vi "Machs1-11-15.vi"(0 "Heizen?Mach1":bool, 1 "Heizen?Mach2":bool, 2 "PIDMach1":T1 {"proportional gain (Kc)" format="%.11g"; "integral gain (Kc*Ts/Ti)" format="%.11g"; "derivative gain (Kc*Td/Ts)" format="%.11g"}, 3 "PIDMach2":T1 {"proportional gain (Kc)" format="%.11g"; "integral gain (Kc*Ts/Ti)" format="%.11g"; "derivative gain (Kc*Td/Ts)" format="%.11g"}, 4 "Umax[V]Mach1":fxp<+/-,16,4> format="%.14g", 5 "Umax[V]Mach2":fxp<+/-,16,4> format="%.14g", 6 "USetp[V]Mach1":fxp<+/-,16,4> format="%.14g", 7 "USetp[V]Mach2":fxp<+/-,16,4> format="%.14g", 10 "Per[us]Mach":u16 caption="Periode Mach [us]", 11 "Mach1maxHigh":u16, 12 "vor der Messung [us]Mach":u16=200, 14 "wie viele Messwerte?Mach":u16, 15 "Mach2High?":bool, 16 "Abstand zwischen Messungen [us]Mach":u16 caption="Abstand zwischen Messungen Mach [us]", 17 "Mach2High":u16) -> (20 "U[V]Mach1":fxp<+/-,16,4> format="%.25g", 21 "U[V]Mach2":fxp<+/-,16,4> format="%.25g", 23 "Mach1maxHigh":u16, 26 "Mach2High?":bool, 27 "Mach2High":u16)   [LabVIEW 2010]
uses:
  <vilib>/eio/EIONode/EIONode.xnode
  <vilib>/rvi/eio/nirviEIOImplementation/nirviEIOImplementation.xnode
  <vilib>/rvi/eio/common/nirviEmuClasses.ctl
  <vilib>/rvi/FXPMathLib/FxpAdd/XNode/nifxpmath_Add.xnode
  <vilib>/rvi/FXPMathLib/FxpAdd/subVIs/nifxpmath_Add_SimConfig.ctl
  <vilib>/fxp/LVFixedPointQuantizationPolicyTypeDef.ctl
  <vilib>/fxp/LVFixedPointOverflowPolicyTypeDef.ctl
  <vilib>/rvi/FXPMathLib/FxpDiv/XNode/nifxpmath_Div.xnode
  <vilib>/rvi/FXPMathLib/FxpDiv/subVIs/nifxpmath_Div_SimConfig.ctl
  <vilib>/rvi/FXPMathLib/FxpMul/XNode/nifxpmath_Multiplier.xnode
  <vilib>/rvi/FXPMathLib/FxpMul/subVIs/nifxpmath_Mul_SimConfig.ctl
  <vilib>/rvi/FXPMathLib/FxpSqrt/XNode/nifxpmath_Sqrt.xnode
  <vilib>/rvi/FXPMathLib/FxpSqrt/subVIs/nifxpmath_Sqrt_SimConfig.ctl
  <vilib>/rvi/FXPMathLib/FxpConvert/XNode/nifxpmath_Convert.xnode
  <vilib>/rvi/FXPMathLib/FxpConvert/subVIs/nifxpmath_Convert_SimConfig.ctl
  <vilib>/addons/control/pid/fpga.llb/XNode/niFpgaPID.xnode
  <vilib>/rvi/eio/common/nirviEmuTemplateMethod_noerrors.vi
  <vilib>/rvi/FXPMathLib/FxpAdd/simVIs/DllFxpAddTemp_sub.vi
  <vilib>/rvi/FXPMathLib/FxpDiv/simVIs/DllFxpDivTemp_sub.vi
  <vilib>/rvi/FXPMathLib/FxpMul/simVIs/DllFxpMulTemp_sub.vi
  <vilib>/rvi/FXPMathLib/FxpSqrt/simVIs/DllSqrtTemp_sub.vi
  <vilib>/rvi/FXPMathLib/FxpConvert/simVIs/DllFxpConvertTemp_sub.vi
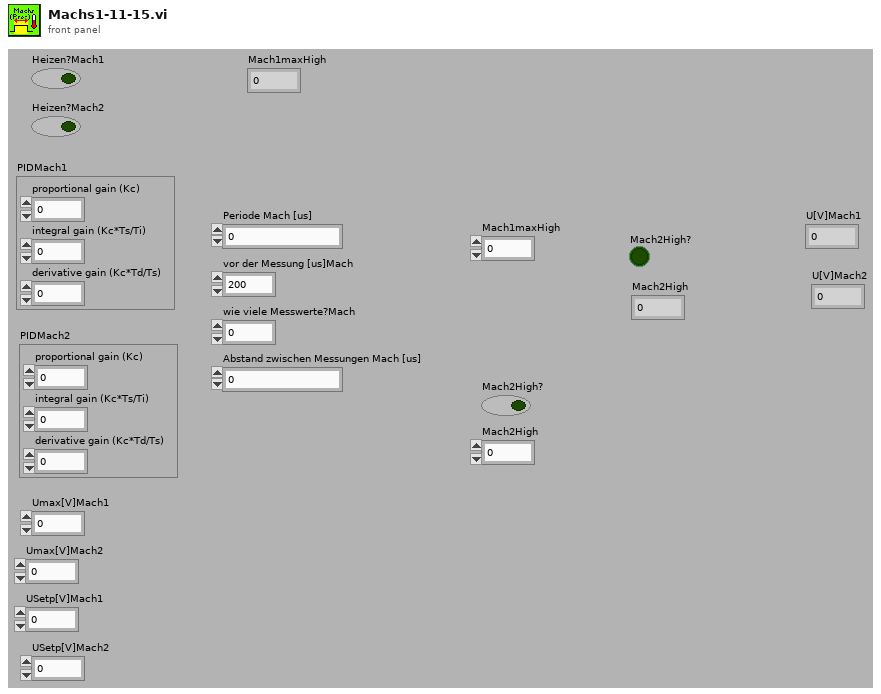
[diagram p1: front panel]
types:
  T1 = cluster{"proportional gain (Kc)":fxp<+/-,16,8>, "integral gain (Kc*Ts/Ti)":fxp<+/-,16,8>, "derivative gain (Kc*Td/Ts)":fxp<+/-,16,8>}
  T2 = cluster{"output high":fxp<+/-,16,4>, "output low":fxp<+/-,16,4>}
  T3 = typedef "nirviEmuClasses.ctl" = enum16{"IO Read", "IO Write", "Method", "Property Read", "Property Write"}
  T4 = cluster{"proportional gain (Kc)":i16, "integral gain (Kc*Ts/Ti)":i16, "derivative gain (Kc*Td/Ts)":i16}
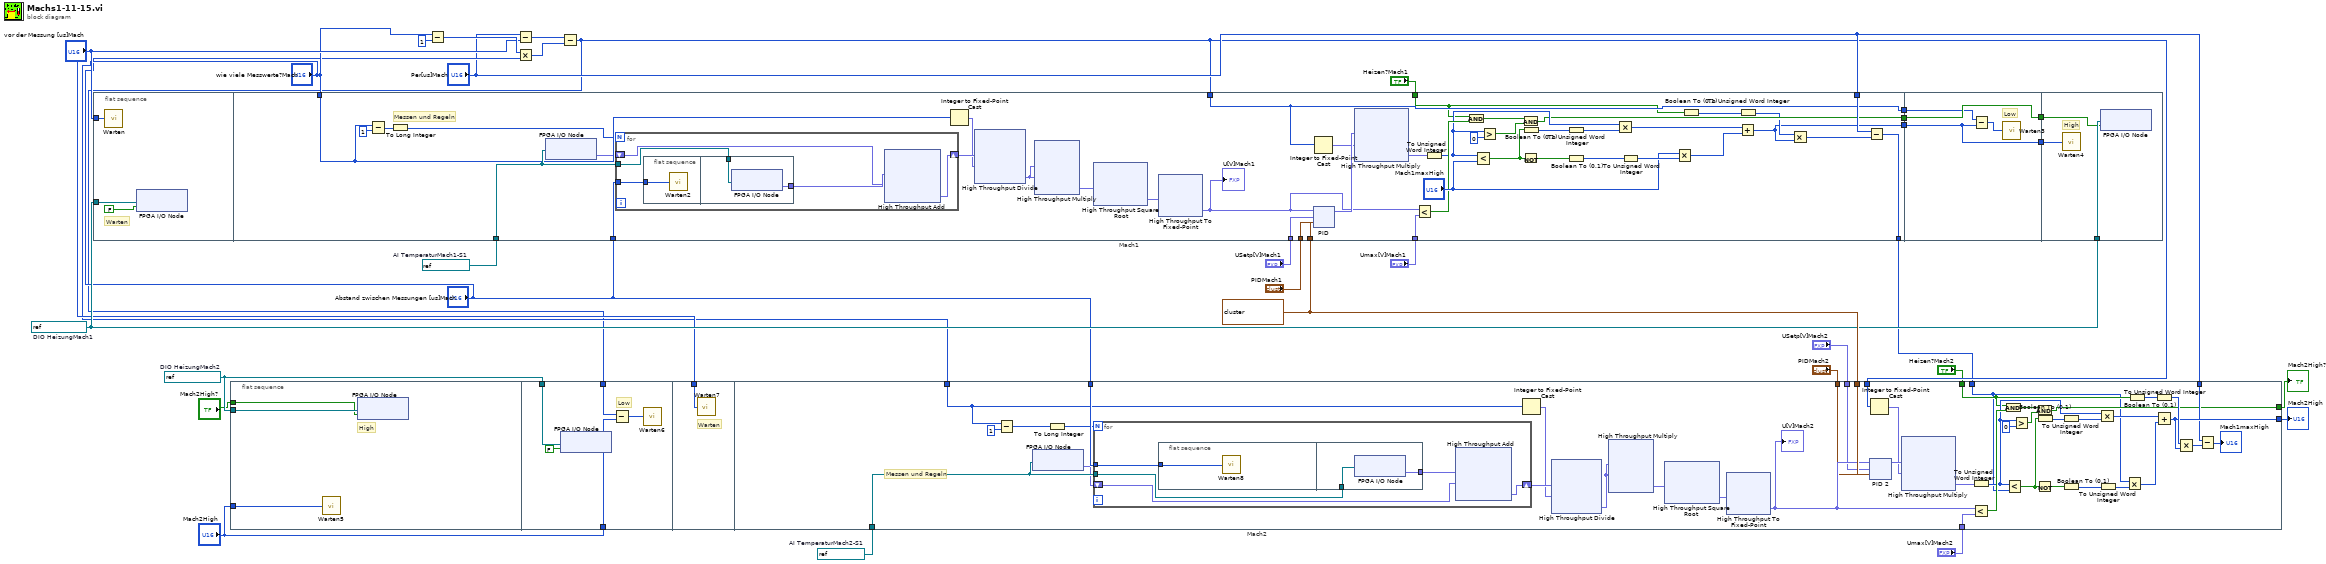
[diagram p0: block diagram]
diagram:
  w23 = refnum<k21> "Mod6/DIO22"  # DIO HeizungMach2
  w24 = refnum<k21> "Mod1/AI4"  # AI TemperaturMach2-S1
  w25 = refnum<k21> "Mod1/AI3"  # AI TemperaturMach1-S1
  w26 = refnum<k21> "Mod6/DIO23"  # DIO HeizungMach1
  w27 = T2 {"output high"=1.0, "output low"=0.0} ("output range")
  n1 = flat-sequence "Mach1" {
    tunnel: "vor der Messung [us]Mach" -> [w35]
    tunnel: w26 -> [w34]
    tunnel: w25 -> [w88]
    tunnel: "Abstand zwischen Messungen [us]Mach" -> [w84]
    tunnel: "wie viele Messwerte?Mach" -> [w86]
    tunnel: "Per[us]Mach" -> [w69]
    tunnel: [w60] -> w32
    tunnel: [w63] -> w31
    tunnel: [w58] -> w30
    tunnel: w10 -> [w58]
    tunnel: w27 -> [w57]
    tunnel: "Umax[V]Mach1" -> [w52]
    tunnel: "USetp[V]Mach1" -> [w51]
    tunnel: "Heizen?Mach1" -> [w50]
    tunnel: "PIDMach1" -> [w49]
    tunnel: [w48] -> w1
    tunnel: [w335] -> w29
    tunnel: w32 -> [w335]
    tunnel: [w336] -> w28
    tunnel: w31 -> [w336]
    tunnel: w30 -> [w334]
    tunnel: w26 -> [w339]
    tunnel: w29 -> [w338]
    tunnel: w28 -> [w337]
    frame #0 {
      # "Warten"
      n2 = call "Warten"("Count(uSec)"=w35) -> ()  [unwired: 1 out]
      n3 = xnode "FPGA I/O Node"("I/O Item"=FALSE, "FPGA I/O In"=w34) -> ()  [unwired: 1 out]
    }
    frame #1 {
      # "Messen und Regeln"
      n4 = Subtract(x=w86, y=u16 1) -> (x-y=w83:u16)
      n5 = To Long Integer(number=w83) -> (32bit integer=w82:i32)
      n6 = xnode "FPGA I/O Node"("FPGA I/O In"=w88) -> ("I/O Item"=w47:fxp<+/-,26,5>)  [unwired: 1 out]
      n7 = for {
        N: w82 -> [_]
        shift-right: [w230] -> w87
        shift-left: w47 -> [w231]
        tunnel: w84 -> [w234]
        tunnel: w88 -> [w233]
        n8 = flat-sequence {
          tunnel: w234 -> [w265]
          tunnel: w233 -> [w267]
          tunnel: [w266] -> w232
          frame #0 {
            n9 = call "Warten2"("Count(uSec)"=w265) -> ()  [unwired: 1 out]
          }
          frame #1 {
            n10 = xnode "FPGA I/O Node"("FPGA I/O In"=w267) -> ("I/O Item"=w266:fxp<+/-,26,5>)  [unwired: 1 out]
          }
        }
        n11 = xnode "High Throughput Add"("x"=w232, "y"=w231) -> ("x+y"=w230:fxp<+/-,32,11>)
      }
      n12 = Integer to Fixed-Point Cast ("Integer in Festkomma umwandeln")(integer=w86) -> (fixed-point=w85:fxp<+/-,8,8>)  [unwired: 1 in]
      n13 = xnode "High Throughput Divide"("x"=w87, "y"=w85) -> ("x/y"=w56:fxp<+/-,16,4>)
      n14 = xnode "High Throughput Multiply"("x"=w56, "y"=w56) -> ("x*y"=w55:fxp<+,32,8>)
      n15 = xnode "High Throughput Square Root"("x"=w55) -> ("sqrt(x)"=w54:fxp<+,16,4>)
      n16 = xnode "High Throughput To Fixed-Point"("x"=w54) -> ("y"=w53:fxp<+/-,16,4>)
      "U[V]Mach1" <- w53
      n17 = xnode ("PID")("process variable"=w53, "setpoint"=w51, "PID gains"=w49, "output range"=w57) -> ("output"=w81:fxp<+/-,16,4>)  [unwired: 1 in]
      n18 = Integer to Fixed-Point Cast ("Integer in Festkomma umwandeln")(integer=w58) -> (fixed-point=w80:fxp<+,16,16>)  [unwired: 1 in]
      n19 = xnode "High Throughput Multiply"("x"=w81, "y"=w80) -> ("x*y"=w79:fxp<+/-,16,16>)
      n20 = Less?(x=w53, y=w52) -> (x < y?=w68:bool)
      n21 = To Unsigned Word Integer(number=w79) -> (unsigned 16bit integer=w67:u16)
      n22 = And(x=w50, y=w68) -> (x .and. y?=w65:bool)
      n23 = Less?(x=w67, y="Mach1maxHigh") -> (x < y?=w74:bool)
      n24 = Greater?(x=w67, y=u16 0) -> (0:w64:bool)
      n25 = And(x=w65, y=w64) -> (x .and. y?=w63:bool)
      n26 = Boolean To (0,1)(Boolean=w74) -> (0, 1=w78:i16)
      n27 = Not(x=w74) -> (.not. x?=w73:bool)
      n28 = To Unsigned Word Integer(number=w78) -> (unsigned 16bit integer=w77:u16)
      n29 = Boolean To (0,1)(Boolean=w73) -> (0, 1=w76:i16)
      n30 = Multiply(x=w67, y=w77) -> (x*y=w71:u16)
      n31 = To Unsigned Word Integer(number=w76) -> (unsigned 16bit integer=w75:u16)
      n32 = Multiply(x="Mach1maxHigh", y=w75) -> (x*y=w70:u16)
      n33 = Boolean To (0,1)(Boolean=w50) -> (0, 1=w62:i16)
      n34 = To Unsigned Word Integer(number=w62) -> (unsigned 16bit integer=w61:u16)
      n35 = Add(x=w71, y=w70) -> (x+y=w60:u16)
      n36 = Multiply(x=w61, y=w60) -> (x*y=w59:u16)
      n37 = Subtract(x=w69, y=w59) -> (x-y=w48:u16)
    }
    frame #2 {
      # "Low"
      n38 = Subtract(x=w334, y=w335) -> (x-y=w333:u16)
      n39 = call "Warten3"("Count(uSec)"=w333) -> ()  [unwired: 1 out]
    }
    frame #3 {
      # "High"
      n40 = call "Warten4"("Count(uSec)"=w338) -> ()  [unwired: 1 out]
      n41 = xnode "FPGA I/O Node"("I/O Item"=w337, "FPGA I/O In"=w339) -> ()  [unwired: 1 out]
    }
  }
  n42 = flat-sequence "Mach2" {
    tunnel: "Mach2High" -> [w351]
    tunnel: w23 -> [w353]
    tunnel: "Mach2High?" -> [w352]
    tunnel: w23 -> [w369]
    tunnel: w10 -> [w367]
    tunnel: "Mach2High" -> [w366]
    tunnel: "vor der Messung [us]Mach" -> [w381]
    tunnel: w24 -> [w423]
    tunnel: "Abstand zwischen Messungen [us]Mach" -> [w424]
    tunnel: "wie viele Messwerte?Mach" -> [w419]
    tunnel: w27 -> [w415]
    tunnel: w10 -> [w400]
    tunnel: [w401] -> w19
    tunnel: "Per[us]Mach" -> [w398]
    tunnel: [w393] -> w20
    tunnel: "USetp[V]Mach2" -> [w388]
    tunnel: "PIDMach2" -> [w387]
    tunnel: "Umax[V]Mach2" -> [w386]
    tunnel: "Heizen?Mach2" -> [w385]
    tunnel: w1 -> [w383]
    frame #0 {
      # "High"
      n43 = call "Warten5"("Count(uSec)"=w351) -> ()  [unwired: 1 out]
      n44 = xnode "FPGA I/O Node"("I/O Item"=w352, "FPGA I/O In"=w353) -> ()  [unwired: 1 out]
    }
    frame #1 {
      # "Low"
      n45 = xnode "FPGA I/O Node"("I/O Item"=FALSE, "FPGA I/O In"=w369) -> ()  [unwired: 1 out]
      n46 = Subtract(x=w367, y=w366) -> (x-y=w365:u16)
      n47 = call "Warten6"("Count(uSec)"=w365) -> ()  [unwired: 1 out]
    }
    frame #2 {
      # "Warten"
      n48 = call "Warten7"("Count(uSec)"=w381) -> ()  [unwired: 1 out]
    }
    frame #3 {
      # "Messen und Regeln"
      n49 = Subtract(x=w419, y=u16 1) -> (x-y=w421:u16)
      n50 = xnode "FPGA I/O Node"("FPGA I/O In"=w423) -> ("I/O Item"=w382:fxp<+/-,26,5>)  [unwired: 1 out]
      n51 = To Long Integer(number=w421) -> (32bit integer=w420:i32)
      n52 = for {
        N: w420 -> [_]
        shift-right: [w592] -> w418
        shift-left: w382 -> [w593]
        tunnel: w424 -> [w596]
        tunnel: w423 -> [w595]
        n53 = flat-sequence {
          tunnel: w596 -> [w627]
          tunnel: w595 -> [w629]
          tunnel: [w628] -> w594
          frame #0 {
            n54 = call "Warten8"("Count(uSec)"=w627) -> ()  [unwired: 1 out]
          }
          frame #1 {
            n55 = xnode "FPGA I/O Node"("FPGA I/O In"=w629) -> ("I/O Item"=w628:fxp<+/-,26,5>)  [unwired: 1 out]
          }
        }
        n56 = xnode "High Throughput Add"("x"=w594, "y"=w593) -> ("x+y"=w592:fxp<+/-,32,11>)
      }
      n57 = Integer to Fixed-Point Cast ("Integer in Festkomma umwandeln")(integer=w419) -> (fixed-point=w417:fxp<+/-,8,8>)  [unwired: 1 in]
      n58 = xnode "High Throughput Divide"("x"=w418, "y"=w417) -> ("x/y"=w392:fxp<+/-,16,4>)
      n59 = xnode "High Throughput Multiply"("x"=w392, "y"=w392) -> ("x*y"=w391:fxp<+,32,8>)
      n60 = xnode "High Throughput Square Root"("x"=w391) -> ("sqrt(x)"=w390:fxp<+,16,4>)
      n61 = xnode "High Throughput To Fixed-Point"("x"=w390) -> ("y"=w389:fxp<+/-,16,4>)
      "U[V]Mach2" <- w389
      n62 = xnode ("PID 2")("process variable"=w389, "setpoint"=w388, "PID gains"=w387, "output range"=w415) -> ("output"=w414:fxp<+/-,16,4>)  [unwired: 1 in]
      n63 = Integer to Fixed-Point Cast ("Integer in Festkomma umwandeln")(integer=w400) -> (fixed-point=w413:fxp<+,16,16>)  [unwired: 1 in]
      n64 = xnode "High Throughput Multiply"("x"=w414, "y"=w413) -> ("x*y"=w404:fxp<+/-,16,16>)
      n65 = Less?(x=w389, y=w386) -> (x < y?=w416:bool)
      n66 = To Unsigned Word Integer(number=w404) -> (unsigned 16bit integer=w396:u16)
      n67 = And(x=w385, y=w416) -> (x .and. y?=w395:bool)
      n68 = Less?(x=w396, y=w383) -> (x < y?=w408:bool)
      n69 = Greater?(x=w396, y=u16 0) -> (0:w394:bool)
      n70 = And(x=w395, y=w394) -> (x .and. y?=w393:bool)
      n71 = Boolean To (0,1)(Boolean=w408) -> (0, 1=w412:i16)
      n72 = Not(x=w408) -> (.not. x?=w407:bool)
      n73 = To Unsigned Word Integer(number=w412) -> (unsigned 16bit integer=w411:u16)
      n74 = Boolean To (0,1)(Boolean=w407) -> (0, 1=w410:i16)
      n75 = Multiply(x=w396, y=w411) -> (x*y=w406:u16)
      n76 = To Unsigned Word Integer(number=w410) -> (unsigned 16bit integer=w409:u16)
      n77 = Multiply(x=w383, y=w409) -> (x*y=w405:u16)
      n78 = Boolean To (0,1)(Boolean=w385) -> (0, 1=w403:i16)
      n79 = To Unsigned Word Integer(number=w403) -> (unsigned 16bit integer=w402:u16)
      n80 = Add(x=w406, y=w405) -> (x+y=w401:u16)
      n81 = Multiply(x=w402, y=w401) -> (x*y=w399:u16)
      n82 = Subtract(x=w398, y=w399) -> (x-y=→"Mach1maxHigh":u16)
    }
  }
  n83 = Subtract(x="wie viele Messwerte?Mach", y=u16 1) -> (x-y=w17:u16)
  n84 = Subtract(x="Per[us]Mach", y="vor der Messung [us]Mach") -> (x-y=w16:u16)
  n85 = Multiply(x=w17, y="Abstand zwischen Messungen [us]Mach") -> (x*y=w15:u16)
  n86 = Subtract(x=w16, y=w15) -> (x-y=w10:u16)
  "Mach2High?" <- w20
  "Mach2High" <- w19
